vi "DSF.Engine.Memory.Cache.Create.vi"(8 "error in (no error)":errorcluster, 10 "Transfers":refnum<class "DSF.Engine.Transfer.lvclass">[](array[class]), 11 "Transfers Groups":refnum<class "DSF.Engine.Transfer Group.lvclass">[](array[class])) -> (0 "error out":errorcluster, 3 "Cache out":refnum<class "DSF.Engine.Memory.Cache.lvclass">)   [LabVIEW 2017, in "DSF.Engine.lvlib" / "DSF.Engine.Memory.Cache.lvclass"]
uses:
  DSF.Engine.Memory.Cache.lvclass
  Transfer/DSF.Engine.Transfer.lvclass
  Transfer/DSF.Engine.Transfer Group.lvclass
  DSF.Engine.Memory.Cache.lvclass/DSF.Engine.Memory.Cache.ctl
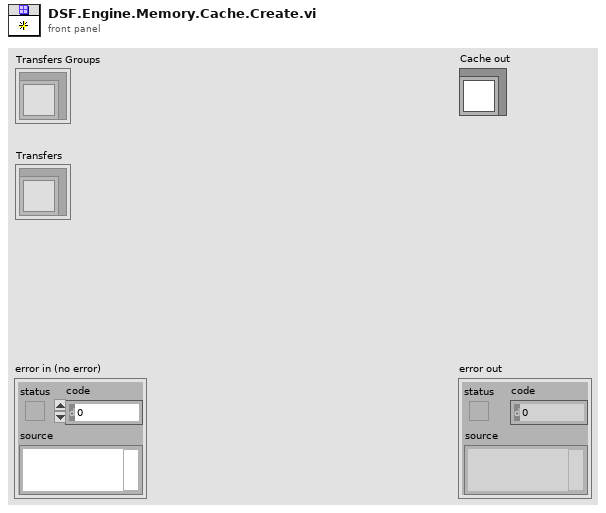
[diagram p1: front panel]
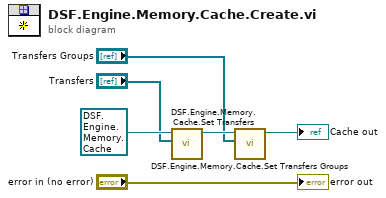
[diagram p0: block diagram]
diagram:
  n1 = call "DSF.Engine.Memory.Cache.Set Transfers.vi"("Transfers"="Transfers", "Cache in"=refnum<class "DSF.Engine.Memory.Cache.lvclass"> refnum) -> ("Cache out"=w4:refnum<class "DSF.Engine.Memory.Cache.lvclass">)  [unwired: 9 in]
  n2 = call "DSF.Engine.Memory.Cache.Set Transfers Groups.vi"("Transfers Groups"="Transfers Groups", "Cache in"=w4) -> ("Cache out"=→"Cache out":refnum<class "DSF.Engine.Memory.Cache.lvclass">)  [unwired: 9 in]
  "error out" <- "error in (no error)"
